vi "Demo.vi"(8 "error in (no error)":errorcluster, 11 "PythonPlotter in":refnum<class "PythonPlotter.lvclass">) -> (0 "error out":errorcluster, 3 "PythonPlotter out":refnum<class "PythonPlotter.lvclass">)   [LabVIEW 2024, in "PythonPlotter.lvclass"]
uses:
  PythonPlotter.lvclass
  #ColormapConfig.ctl
  PythonPlotter.lvclass/PythonPlotter.ctl
  <vilib>/Analysis/1siggen.llb/Ramp Pattern by Samples.vi
  <vilib>/Analysis/NI_AALBase.lvlib
  <vilib>/measure/NI_MABase.lvlib
panel:
  in  "Env path":path=path "C:/Users/bogum/OneDrive/Dokumenty/Git/LabVIEW Python Ploter/.venv"
  in  "module path 2":path=path "C:/Users/bogum/OneDrive/Dokumenty/Git/LabVIEW Python Ploter/LabVIEW_python_ploter.py"
  in  "Colormap Config":T1
  in  "target path":path=path "C:/Users/bogum/OneDrive/Obrazy/test/mapa2.svg"
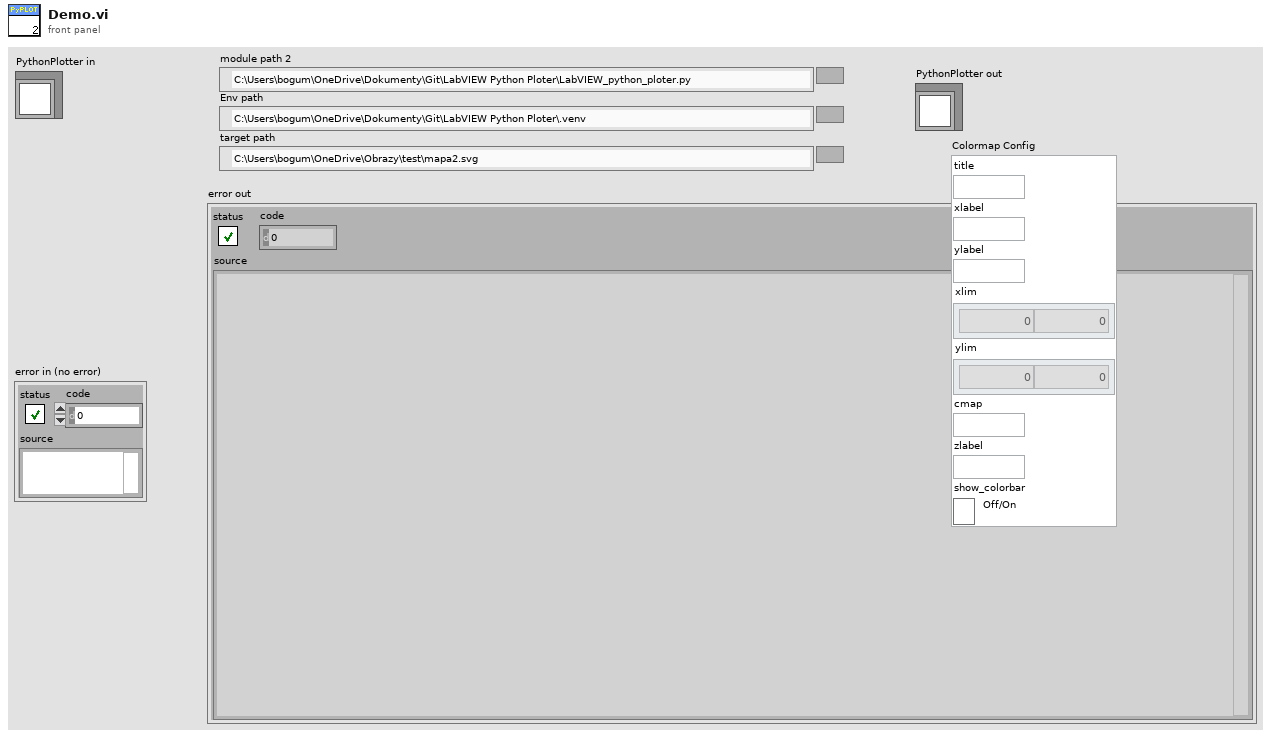
[diagram p1: front panel]
types:
  T1 = typedef "PythonPlotter.lvclass/#ColormapConfig.ctl" = cluster{"title":string, "xlabel":string, "ylabel":string, "xlim":dbl[], "ylim":dbl[], "cmap":string, "zlabel":string, "show_colorbar":bool}
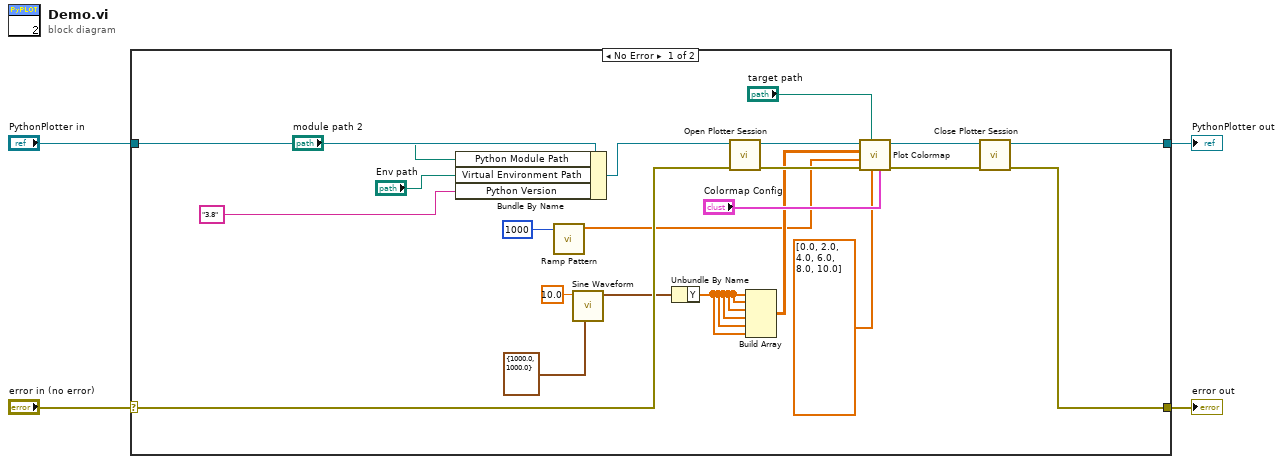
[diagram p0: block diagram]
diagram:
  n1 = case shown="No Error" "error in (no error)" {
    selector: "error in (no error)" -> [w20 w28]
    tunnel: [w19 w28] -> w3
    tunnel: [w22 w27] -> w1
    tunnel: "PythonPlotter in" -> [w26 w27]
    frame No Error {
      n2 = Bundle By Name(cluster=w26, "Python Module Path"="module path 2", "Virtual Environment Path"="Env path", "Python Version"="3.8" ("Python version")) -> (w21:refnum<class "PythonPlotter.lvclass">)
      n3 = call-poly <vilib>:"Ramp Pattern.vi"("samples"=1000) -> ("Ramp Pattern"=w6:dbl[])  [unwired: 9 in, 1 out]
      n4 = call <vilib>:"Sine Waveform.vi"("sampling info"=cluster{"Fs":dbl, "#s":dbl} {"Fs"=1000.0, "#s"=1000.0}, "frequency"=10.0) -> ("signal out"=w15:waveform(dbl))  [unwired: 8 in, 1 out]
      n5 = Unbundle By Name(w15) -> ("Y"=w8:dbl[])
      n6 = call "Open Plotter Session.vi"("error in (no error)"=w20, "PythonPlotter in"=w21) -> ("error out"=w13:errorcluster, "PythonPlotter out"=w12:refnum<class "PythonPlotter.lvclass">)  [unwired: 8 in]
      n7 = Build Array(w8, w8, w8, w8, w8, w8) -> (w7:dbl[][])
      n8 = call "Plot Colormap.vi"("Colormap Config"="Colormap Config", "Y"=dbl[] [0.0, 2.0, 4.0, 6.0, 8.0, 10.0], "target path"="target path", "error in (no error)"=w13, "X"=w6, "Data 2d"=w7, "PythonPlotter in"=w12) -> ("error out"=w14:errorcluster, "PythonPlotter out"=w11:refnum<class "PythonPlotter.lvclass">)  [unwired: 3 in]
      n9 = call "Close Plotter Session.vi"("error in (no error)"=w14, "PythonPlotter in"=w11) -> ("error out"=w19:errorcluster, "PythonPlotter out"=w22:refnum<class "PythonPlotter.lvclass">)  [unwired: 8 in]
    }
    frame Error {
    }
  }
  "error out" <- w3
  "PythonPlotter out" <- w1
